vi "V-Meter Adjust 3706 Measure.vi"(6 "Slot Number":u8=1 min=1 max=6, 7 "error in (no error)":errorcluster, 10 "VISA resource name in":refnum<visa-resource-name>) -> (0 "error out":errorcluster, 3 "VISA resource name out":refnum<visa-resource-name>)   [LabVIEW 2016, in "Hall Effect Library.lvlib"]
uses:
  Hall Effect Library.lvlib
  <instrlib>/Keithley 3706/Keithley 3706.lvlib
panel:
  out "Measurement":dbl
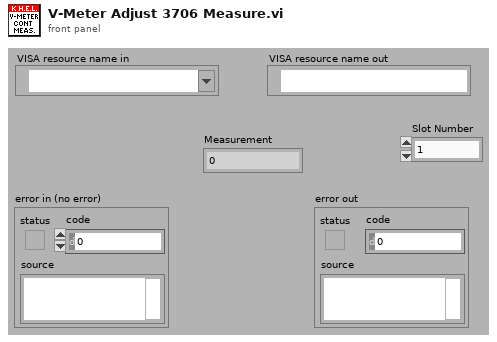
[diagram p1: front panel]
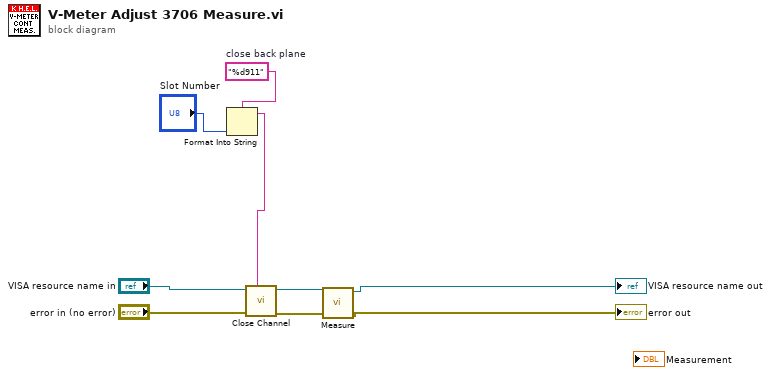
[diagram p0: block diagram]
diagram:
  w8 = "%d911"  # close back plane
  n1 = Format Into String(format string=w8, "Slot Number") -> (resulting string=w5:string)  [unwired: 2 in, 1 out]
  n2 = call <instrlib>:"Close Channel.vi"("Channel List"=w5, "error in (no error)"="error in (no error)", "VISA resource name"="VISA resource name in") -> ("error out"=w3:errorcluster, "VISA resource name out"=w4:refnum<visa-resource-name>)  [unwired: 7 in]
  n3 = call <instrlib>:"Measure.vi"("error in (no error)"=w3, "VISA resource name"=w4) -> ("error out"=→"error out":errorcluster, "VISA resource name out"=→"VISA resource name out":refnum<visa-resource-name>)  [unwired: 7 in, 1 out]
